vi "Event Handle Loop_Pop-out Panel_Set Page Attribute.vi"(8 "error in (no error)":errorcluster, 10 "Pag Attribute":T1, 11 "QTab Class in":refnum<class "QTab Class.lvclass">) -> (0 "error out":errorcluster, 3 "QTab Class out":refnum<class "QTab Class.lvclass">)   [LabVIEW 2020, in "QTab.lvlib" / "QTab Class.lvclass"]
uses:
  QTab Class.lvclass
  Pag Attribute.ctl
  QTab Class.lvclass/QTab Class.ctl
  Command.ctl
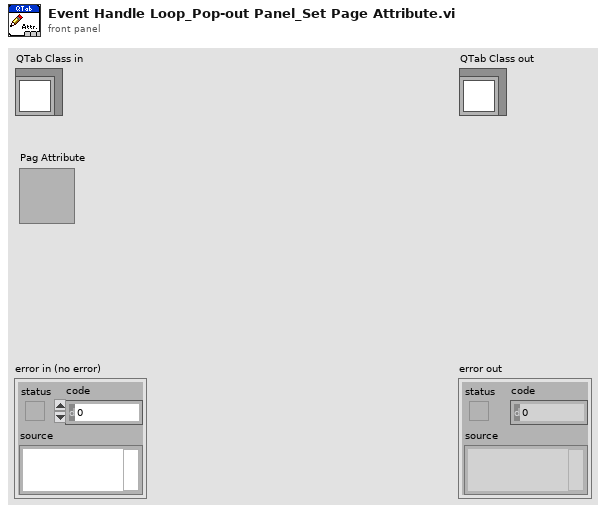
[diagram p1: front panel]
types:
  T1 = typedef "QTab.lvlib/QTab Class.lvclass/Pag Attribute.ctl" = cluster{"VI Refnum":refnum<vi>, "Page Name":string, "Closeable":bool, "Draggable":bool, "Pop-Out":bool}
  T2 = typedef "QTab.lvlib/QTab Class.lvclass/Command.ctl" = enum16{"Startup", "Add Page", "Close All Page", "Set Page Attribute", "Pop-out", "Merage", "Insert", "Stop"}
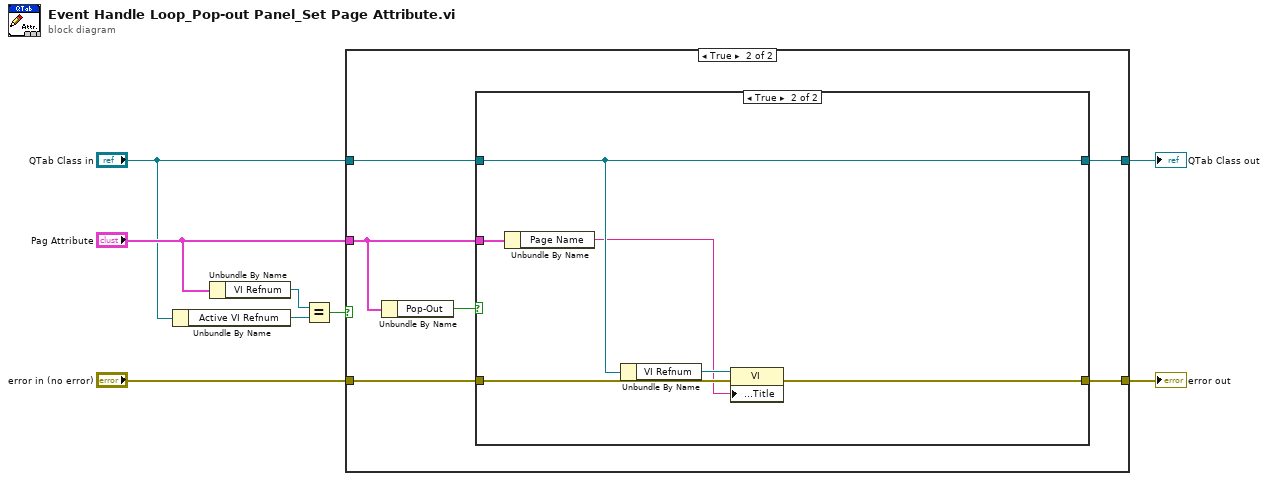
[diagram p0: block diagram]
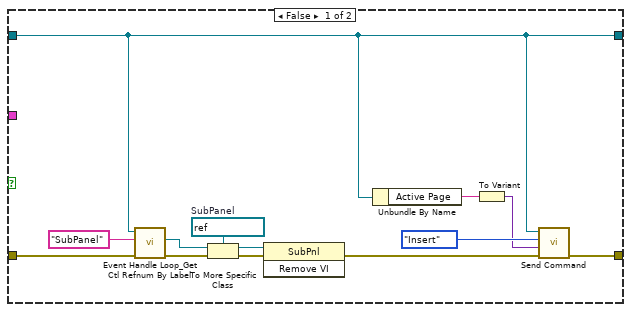
[diagram p3: hidden frame]
diagram:
  n1 = Unbundle By Name("QTab Class in") -> ("Active VI Refnum"=w8:refnum<vi>)
  n2 = Unbundle By Name("Pag Attribute") -> ("VI Refnum"=w7:refnum<vi>)
  n3 = Equal?(x=w7, y=w8) -> (x = y?=w6:bool)
  n4 = case shown="True" w6 {
    tunnel: "Pag Attribute" -> [_ w15]
    tunnel: "QTab Class in" -> [w10 w14]
    tunnel: [w10 w13] -> w5
    tunnel: "error in (no error)" -> [w9 w12]
    tunnel: [w9 w11] -> w1
    frame False {
    }
    frame True {
      n5 = Unbundle By Name(w15) -> ("Pop-Out"=w16:bool)
      n6 = case shown="True" w16 {
        tunnel: w15 -> [_ w31]
        tunnel: w14 -> [w17 w35]
        tunnel: [w17 w35] -> w13
        tunnel: w12 -> [w23 w34]
        tunnel: [w18 w32] -> w11
        frame False {
          w26 = refnum<vi> refnum  # SubPanel
          n7 = call "Event Handle Loop_Get Ctl Refnum By Label.vi"("error in (no error)"=w23, "Label"="SubPanel", "QTab Class in"=w17) -> ("error out"=w28:errorcluster, "Ctl Refnum"=w27:refnum<vi>)  [unwired: 6 in, 1 out]
          n8 = To More Specific Class(target class=w26, reference=w27, error in=w28) -> (specific class reference=w24:refnum<vi>, error out=w25:errorcluster)
          n9 = invoke class="SubPnl" method="Remove VI"(reference=w24, error in=w25) -> (error out=w19:errorcluster)  [unwired: 1 in, 2 out]
          n10 = Unbundle By Name(w17) -> ("Active Page"=w21:string)
          n11 = To Variant(anything=w21) -> (Variant=w20:variant)
          n12 = call "Send Command.vi"("error in (no error)"=w19, "Data"=w20, "Command"=Command."Insert", "QTab Class in"=w17) -> ("error out"=w18:errorcluster)  [unwired: 6 in, 1 out]
        }
        frame True {
          n13 = Unbundle By Name(w31) -> ("Page Name"=w30:string)
          n14 = Unbundle By Name(w35) -> ("VI Refnum"=w33:refnum<vi>)
          n15 = property class="VI"(reference=w33, error in=w34, "Front Panel.Title"=w30) -> (error out=w32:errorcluster)  [unwired: 1 out]
        }
      }
    }
  }
  "error out" <- w1
  "QTab Class out" <- w5
